vi "Find all visa.vi"(8 "error in":errorcluster) -> (0 "error out":errorcluster, 1 "# of Address Found":i32, 2 "Cancelled?":bool, 3 "element":string)   [LabVIEW 2013]
uses:
  States of Find all.ctl
  Display Panel/Display Panel.lvlib
  Universal Power Meter/Universal Power Meter class/Universal Power Meter.lvclass
  Generic Instrument/Generic Instrument.lvclass
panel:
  out "SMALL i":i32
  out "big I":i32
  out "Array":errorcluster[](array[cluster])
  out "Current State":T1=enum."Searching"
  in  "Retry":bool
  in  "Stop Button":bool
  in  "Card to Start":u16(ring) items=["YOKOGAWA WT500 @address: GPIB0::5::INSTR"]
  in  "Cancel Button":bool
  out "Boolean":bool
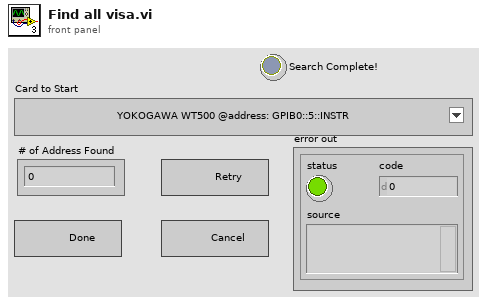
[diagram p1: front panel]
types:
  T1 = typedef "States of Find all.ctl" = enum16{"Idle", "Done", "Searching"}
  T2 = enum8{"Enabled", "Disabled", "Disabled and Grayed Out"}
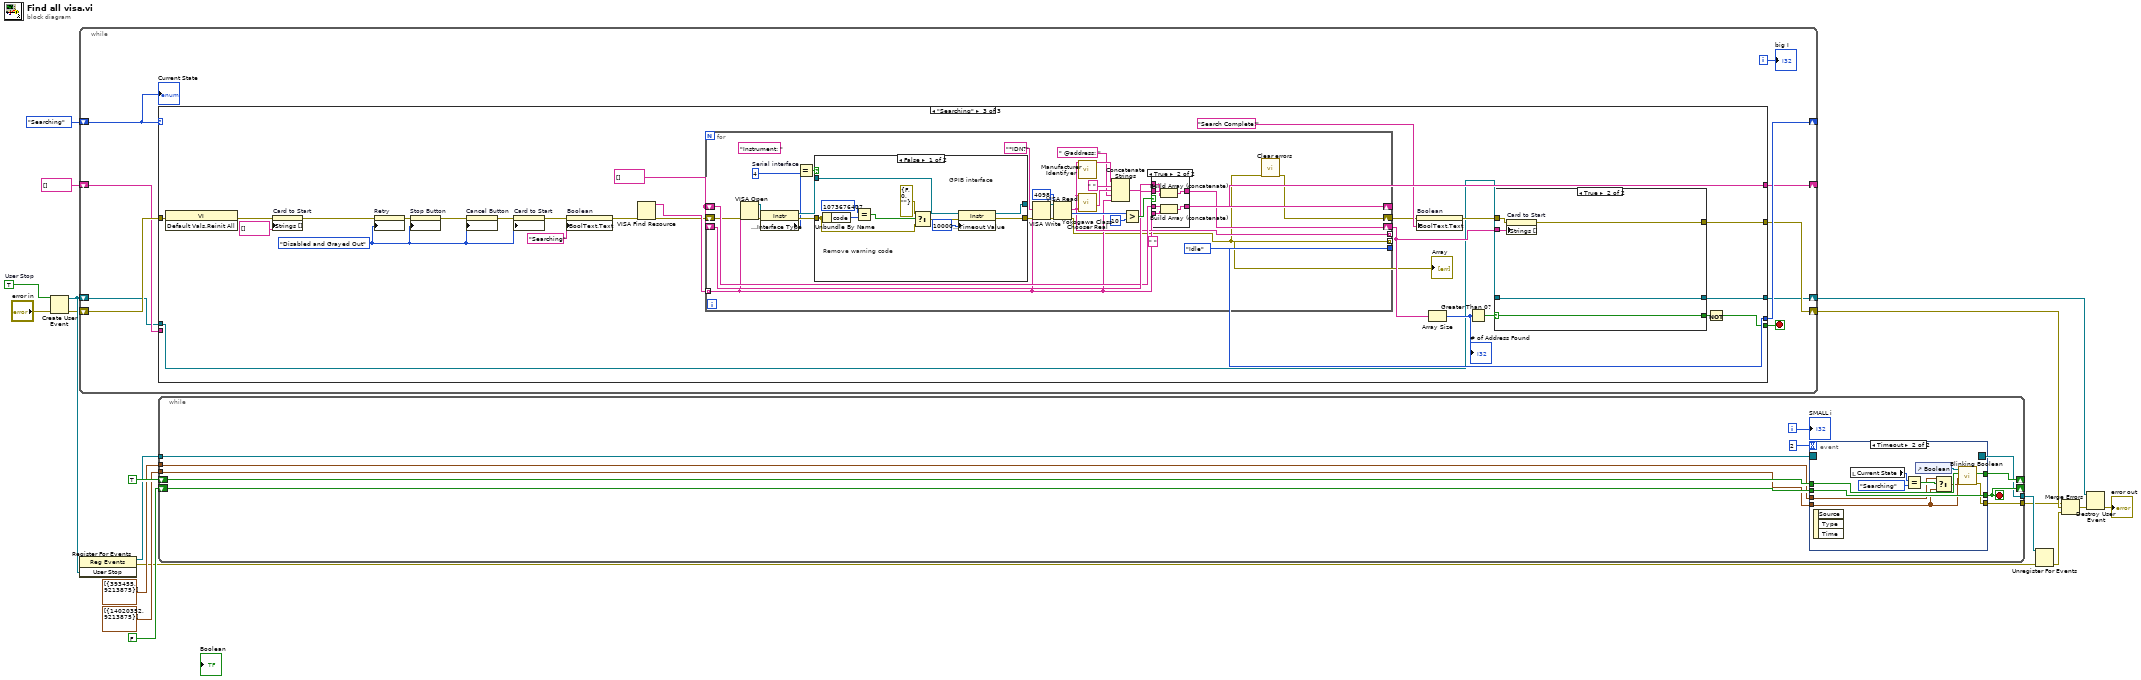
[diagram p0: block diagram]
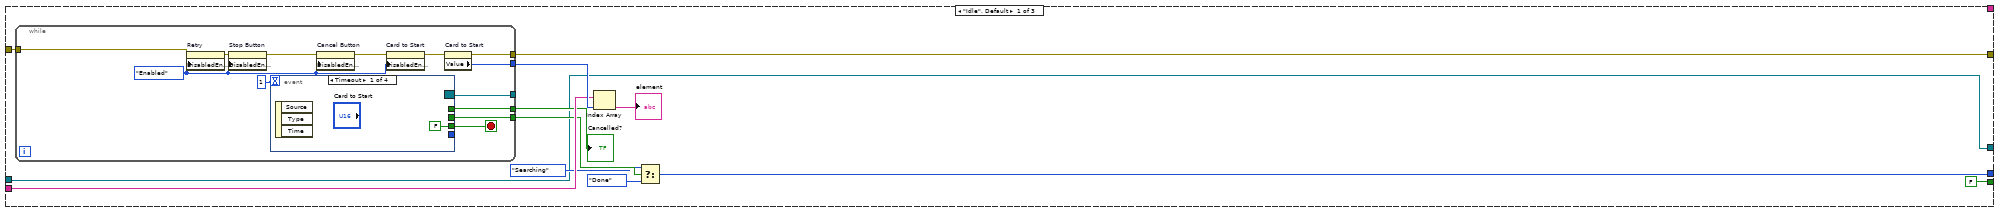
[diagram p2: hidden frame]
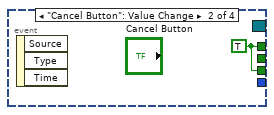
[diagram p3: hidden frame]
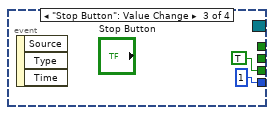
[diagram p4: hidden frame]
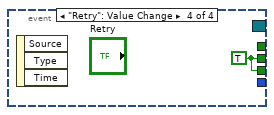
[diagram p5: hidden frame]
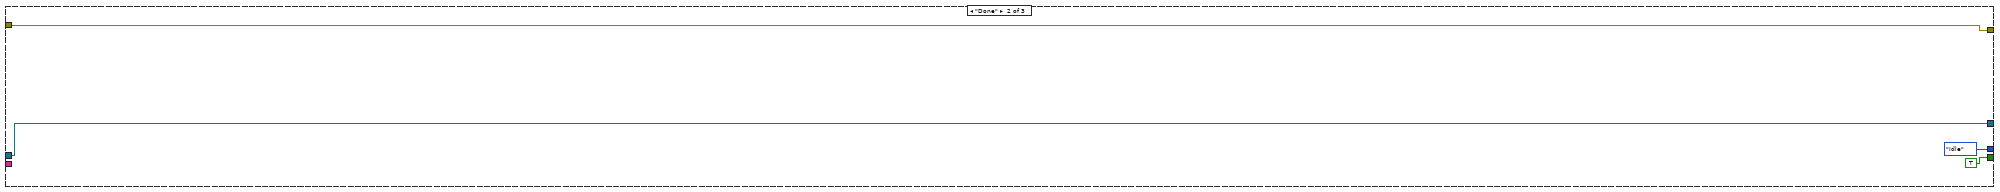
[diagram p6: hidden frame]
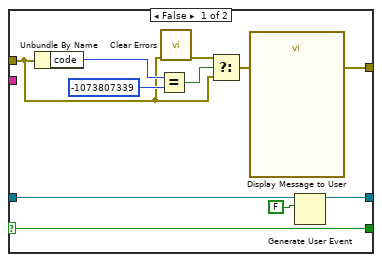
[diagram p7: hidden frame]
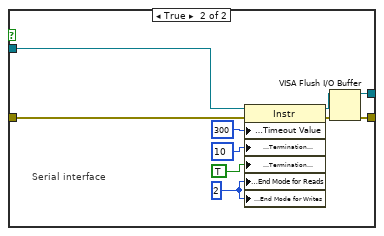
[diagram p8: hidden frame]
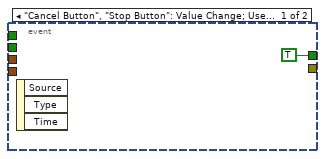
[diagram p10: hidden frame]
diagram:
  w13 = TRUE  # User Stop
  n1 = Create User Event(user event datatype=w13, error in="error in") -> (user event=w9:refnum<user-event>, error out=w2:errorcluster)
  n2 = while {
    shift-right: [w28] -> _
    shift-left: States_of_Find_all."Searching" ("Enum") -> [w29]
    shift-right: [w23] -> w8
    shift-left: w2 -> [w26]
    shift-right: [w25] -> _
    shift-left: string[] [] -> [w24]
    shift-right: [w21] -> w6
    shift-left: w9 -> [w22]
    i -> [w20]
    stop <- w27 stop-if-true
    n3 = case shown="\"Searching\"" w29 {
      tunnel: [w31 States_of_Find_all."Idle" ("Enum") w79] -> w28
      tunnel: [FALSE TRUE w69] -> w27
      tunnel: [w36 w61 w86] -> w23
      tunnel: w26 -> [w37 w61 w85]
      tunnel: [_ _ w84] -> w25
      tunnel: w24 -> [w39 _ _]
      tunnel: w22 -> [w30 w60 w68]
      tunnel: [w30 w60 w67] -> w21
      frame "Idle", Default {
        n4 = while {
          tunnel: [w53] -> _
          tunnel: [w51] -> w40
          tunnel: w37 -> [w44]
          tunnel: [w50] -> w36
          tunnel: [w49] -> w35
          tunnel: [w48] -> w34
          stop <- w54 stop-if-true
          w42 = T2."Enabled" ("Disabled")
          n5 = property on="Retry" class="Bool"(error in=w44, "DisabledEnum"=w42) -> (error out=w47:errorcluster)  [unwired: 1 in, 1 out]
          n6 = property on="Stop Button" class="Bool"(error in=w47, "DisabledEnum"=w42) -> (error out=w46:errorcluster)  [unwired: 1 in, 1 out]
          n7 = event shown="[0] Timeout" {
            selector: _ -> [_ _ _ _]
            dyn-events: [_ _ _ _] -> w53
            timeout: 1 -> [_ _ _ _]
            tunnel: [FALSE ("Stop Button") w56 TRUE ("Stop Button") w59] -> w54
            tunnel: [_ _ u16 1 ("Card to Start") _] -> _
            tunnel: [_ w56 _ _] -> w49
            tunnel: [_ _ _ w59] -> w48
            event Timeout {
              n8 = event-data() -> ()  [unwired: 1 in, 3 out]
            }
            event "Cancel Button": Value Change {
              w56 = TRUE ("Stop Button")
              n9 = event-data() -> ()  [unwired: 1 in, 3 out]
            }
            event "Stop Button": Value Change {
              n10 = event-data() -> ()  [unwired: 1 in, 3 out]
            }
            event "Retry": Value Change {
              w59 = TRUE
              n11 = event-data() -> ()  [unwired: 1 in, 3 out]
            }
          }
          n12 = property on="Cancel Button" class="Bool"(error in=w46, "DisabledEnum"=w42) -> (error out=w45:errorcluster)  [unwired: 1 in, 1 out]
          n13 = property on="Card to Start" class="Ring (strict)"(error in=w45, "DisabledEnum"=w42) -> (error out=w43:errorcluster)  [unwired: 1 in, 1 out]
          n14 = property on="Card to Start" class="Ring (strict)"(error in=w43) -> (error out=w50:errorcluster, "Value"=w51:u16)  [unwired: 1 in, 1 out]
        }
        "Cancelled?" <- w35
        n15 = Index Array(array=w39, index=w40) -> (element=→"element":string)
        n16 = Select(t=States_of_Find_all."Searching" ("Enum"), s=w34, f=States_of_Find_all."Done" ("Enum")) -> (s? t:f=w31:T1)
      }
      frame "Done" {
      }
      frame "Searching" {
        w71 = T2."Disabled and Grayed Out" ("Disabled")
        w87 = string[] []
        n17 = invoke class="VI" method="Default Vals.Reinit All"(error in=w85) -> (error out=w81:errorcluster)  [unwired: 2 in, 2 out]
        n18 = property on="Card to Start" class="Ring (strict)"(error in=w81, "Strings []"=string[] []) -> (error out=w73:errorcluster)  [unwired: 1 in, 1 out]
        n19 = property on="Retry" class="Bool"(error in=w73, "DisabledEnum"=w71) -> (error out=w74:errorcluster)  [unwired: 1 in, 1 out]
        n20 = property on="Stop Button" class="Bool"(error in=w74, "DisabledEnum"=w71) -> (error out=w75:errorcluster)  [unwired: 1 in, 1 out]
        n21 = property on="Cancel Button" class="Bool"(error in=w75, "DisabledEnum"=w71) -> (error out=w76:errorcluster)  [unwired: 1 in, 1 out]
        n22 = property on="Card to Start" class="Ring (strict)"(error in=w76, "DisabledEnum"=w71) -> (error out=w72:errorcluster)  [unwired: 1 in, 1 out]
        n23 = property on="Boolean" class="Bool (strict)"(error in=w72, "BoolText.Text"="Searching" ("Boolean Text.Text")) -> (error out=w78:errorcluster)  [unwired: 1 in, 1 out]
        n24 = VISA Find Resource(8:w78) -> (0:w66:errorcluster, 3:w91:string[])  [unwired: 2 in, 1 out]
        n25 = for {
          tunnel: w91 -> [w114] mode=indexing
          shift-right: [w125] -> w90
          shift-left: w87 -> [w132]
          shift-right: [w130] -> w84
          shift-left: w87 -> [w131]
          tunnel: [States_of_Find_all."Idle" ("Enum")] -> w79
          tunnel: [w126] -> _ mode=indexing
          shift-right: [w108] -> w65
          shift-left: w66 -> [w111]
          tunnel: [w109] -> w64 mode=indexing
          w115 = u16 4  # Serial interface
          (unwired) " " ("string")
          (unwired) "Instrument: " ("string")
          n26 = VISA Open(error in (no error)=w111, VISA resource name=w114) -> (VISA resource name=w113:refnum<visa-resource-name>, error out=w112:errorcluster)  [unwired: 3 in]
          n27 = property class="Instr"(reference=w113, error in=w112) -> (reference out=w119:refnum<visa-resource-name>, error out=w118:errorcluster, "Interface Information:Interface Type"=w116:u16)
          n28 = Equal?(x=w116, y=w115) -> (x = y?=w117:bool)
          n29 = case shown="False" w117 {
            tunnel: [w147 w149] -> _
            tunnel: [w146 w148] -> w110
            tunnel: w119 -> [w145 w153]
            tunnel: w118 -> [w140 w152]
            frame False {
              # "GPIB interface"
              # "Remove warning code"
              n30 = Unbundle By Name(w140) -> ("code"=w143:i32)
              n31 = Equal?(x=1073676407, y=w143) -> (x = y?=w141:bool)
              n32 = Select(t=errorcluster {"status"=FALSE, "code"=0, "source"=""}, s=w141, f=w140) -> (s? t:f=w138:errorcluster)
              n33 = property class="Instr"(reference=w145, error in=w138, "General Settings:Timeout Value"=u32 10000 ("Tmo Value")) -> (reference out=w147:refnum<visa-resource-name>, error out=w146:errorcluster)
            }
            frame True {
              w154 = u16 2
              # "Serial interface"
              n34 = property class="Instr"(reference=w153, error in=w152, "General Settings:Timeout Value"=u32 300 ("Tmo Value"), "Message Based Settings:Termination Character"=u8 10, "Message Based Settings:Termination Character Enable"=TRUE, "Serial Settings:End Mode for Reads"=w154, "Serial Settings:End Mode for Writes"=w154) -> (reference out=w151:refnum<visa-resource-name>, error out=w150:errorcluster)
              n35 = VISA Flush I/O Buffer(VISA resource name=w151, error in (no error)=w150) -> (VISA resource name out=w149:refnum<visa-resource-name>, error out=w148:errorcluster)  [unwired: 1 in]
            }
          }
          n36 = VISA Write(VISA resource name=w114, write buffer="*IDN?", error in (no error)=w110) -> (VISA resource name out=w120:refnum<visa-resource-name>, error out=w121:errorcluster)  [unwired: 1 out]
          n37 = VISA Read(VISA resource name=w120, byte count=u32 4098, error in (no error)=w121) -> (read buffer=w126:string, return count=w135:u32, error out=w109:errorcluster)  [unwired: 1 out]
          n38 = call "Manufacturer Identifyer.vi"("Visa In"=w126) -> ("string"=w129:string)  [unwired: 9 in, 1 out]
          n39 = call "Yokogawa Class Chooser Real.vi"("Incoming ID in"=w126) -> ("Model"=w123:string)  [unwired: 8 in, 2 out]
          n40 = Concatenate Strings(w129, " " ("read buffer"), w123, " @address: " ("string"), w114) -> (w128:string)
          n41 = Greater?(x=w135, y=u32 10) -> (0:w134:bool)
          n42 = case shown="True" w134 {
            tunnel: w132 -> [w159 w164]
            tunnel: [w159 w165] -> w125
            tunnel: w131 -> [w158 w163]
            tunnel: [w158 w162] -> w130
            tunnel: w114 -> [_ w161]
            tunnel: w128 -> [_ w160]
            frame False {
            }
            frame True {
              n43 = Build Array (concatenate)(w164, w160) -> (w165:string[])
              n44 = Build Array (concatenate)(w163, w161) -> (w162:string[])
            }
          }
          n45 = call <vilib>:"Clear errors.vi"("error in"=w109) -> ("error out"=w108:errorcluster)  [unwired: 8 in, 2 out]
        }
        "Array" <- w64
        n46 = property on="Boolean" class="Bool (strict)"(error in=w65, "BoolText.Text"="Search Complete!" ("Boolean Text.Text")) -> (error out=w80:errorcluster)  [unwired: 1 in, 1 out]
        n47 = Array Size(array=w90) -> (size(s)=w89:i32)
        "# of Address Found" <- w89
        n48 = Greater Than 0?(x=w89) -> (x > 0?=w88:bool)
        n49 = case shown="True" w88 {
          selector: w88 -> [w95 w104]
          tunnel: w90 -> [_ w107]
          tunnel: [w102 w106] -> w86
          tunnel: w80 -> [w97 w105]
          tunnel: [w95 w104] -> w70
          tunnel: w68 -> [w94 w103]
          tunnel: [w92 w103] -> w67
          frame False {
            n50 = Unbundle By Name(w97) -> ("code"=w101:i32)
            n51 = Equal?(x=w101, y=-1073807339) -> (x = y?=w99:bool)
            n52 = call <vilib>:"Clear Errors.vi"("error in (no error)"=w97) -> ("error out"=w96:errorcluster)  [unwired: 6 in]
            n53 = Select(t=w96, s=w99, f=w97) -> (s? t:f=w98:errorcluster)
            n54 = call "Display Message to User"("error in (no error)"=w98) -> ("error out"=w102:errorcluster)  [unwired: 9 in, 1 out]
            n55 = Generate User Event(user event=w94, event data cluster=FALSE ("event data")) -> (user event out=w92:refnum<user-event>)  [unwired: 2 in, 1 out]
          }
          frame True {
            n56 = property on="Card to Start" class="Ring (strict)"(error in=w105, "Strings []"=w107) -> (error out=w106:errorcluster)  [unwired: 1 in, 1 out]
          }
        }
        n57 = Not(x=w70) -> (.not. x?=w69:bool)
      }
    }
    "Current State" <- w29
    "big I" <- w20
  }
  n58 = register-events(w9) -> (reference out=w12:refnum<event-registration>, error out=w10:errorcluster)  [unwired: 2 in]
  n59 = while {
    shift-right: [w176] -> _
    shift-left: TRUE ("Shift out") -> [w175]
    shift-right: [w173] -> _
    shift-left: FALSE -> [w172]
    tunnel: cluster{u32, u32}[] [{14020352, 9213875}] ("Color 1 (Background, Foreground)") -> [w171]
    tunnel: cluster{u32, u32}[] [{393455, 9213875}] ("Color 2 (Background, Foreground)") -> [w170]
    tunnel: w12 -> [w169]
    tunnel: [w168] -> w11
    tunnel: [w166] -> w1
    i -> [w167]
    stop <- w173 stop-if-true
    n60 = event shown="[1] Timeout" {
      selector: w169 -> [_ _]
      dyn-events: [_ _] -> w168
      timeout: 2 -> [_ _]
      tunnel: [_ w187] -> w176
      tunnel: w175 -> [_ w186]
      tunnel: [TRUE w185] -> w173
      tunnel: w172 -> [_ w185]
      tunnel: w171 -> [_ w180]
      tunnel: w170 -> [_ w181]
      tunnel: [_ w178] -> w166
      event "Cancel Button", "Stop Button": Value Change; User Event {
        n61 = event-data() -> ()  [unwired: 1 in, 3 out]
      }
      event Timeout {
        n62 = event-data() -> ()  [unwired: 1 in, 3 out]
        n63 = local read "Current State"() -> (w184:T1)
        n64 = Equal?(x=w184, y=States_of_Find_all."Searching" ("Enum")) -> (x = y?=w182:bool)
        n65 = control-ref of="Boolean"() -> (w188:refnum<vi>)
        n66 = Select(t=w181, s=w182, f=w180) -> (s? t:f=w179:cluster{u32, u32}[])
        n67 = call "Blinking Boolean.vi"("Color 2 (Background, Foreground)"=w179, "Color 1 (Background, Foreground)"=w180, "Shift in"=w186, "Bool Refnum"=w188) -> ("error out"=w178:errorcluster, "Shift out"=w187:bool)  [unwired: 5 in, 1 out]
      }
    }
    "SMALL i" <- w167
  }
  n68 = Unregister For Events(event registration refnum=w11, error in=w10) -> (error out=w4:errorcluster)
  n69 = Merge Errors(w1, w8, w4) -> (w7:errorcluster)
  n70 = Destroy User Event(user event=w6, error in=w7) -> (error out=→"error out":errorcluster)
